vi "pl1000MaxValue.vi"(8 "error in (no error)":errorcluster, 11 "pl1000 handle":i16) -> (0 "error out":errorcluster, 2 "maxValue":u16, 3 "pl1000 handle out":i16)   [LabVIEW 2016, in "pl1000.lvlib"]
doc: "This function returns the maximum ADC value that the device will return. This value may be different on different models in the PicoLog 1000 Series."
uses:
  pl1000.lvlib
  pl1000.dll
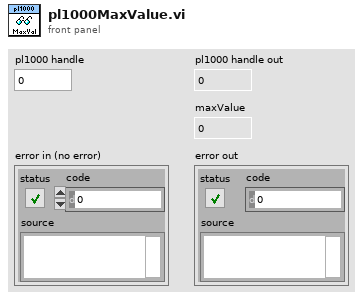
[diagram p1: front panel]
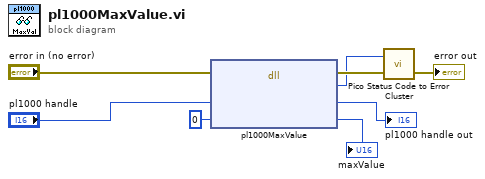
[diagram p0: block diagram]
diagram:
  n1 = dll-call lib="pl1000.dll" fn="pl1000MaxValue"(error in="error in (no error)", "handle"="pl1000 handle", "maxValue"=u16 0) -> (error out=w6:errorcluster, "status"=w5:u32, "handle"=→"pl1000 handle out":i16, "maxValue"=→"maxValue":u16)  [unwired: 2 in, 1 out]
  n2 = call "Pico Status Code to Error Cluster.vi"("error in"=w6, "PICO_STATUS"=w5) -> ("error out"=→"error out":errorcluster)  [unwired: 1 in]
